vi "RSZVB Set Mixer Delay Constant.vi"(8 "error in (no error)":errorcluster {"code" format="%.0x"}, 9 "Constant Delay (0.0 s)":dbl format="%^.3e", 10 "Channel (1)":i32=1, 11 "VISA session":refnum<visa-resource-name>) -> (0 "error out":errorcluster {"code" format="%.0x"}, 3 "dup VISA session":refnum<visa-resource-name>)   [LabVIEW 2011]
doc: "Defines a constant mixer delay value, to be used as a reference for a mixer delay measurement calibration.\n\nRemote-control command(s):\n[SENSe<Ch>:]FREQuency:MDELay:CDELay"
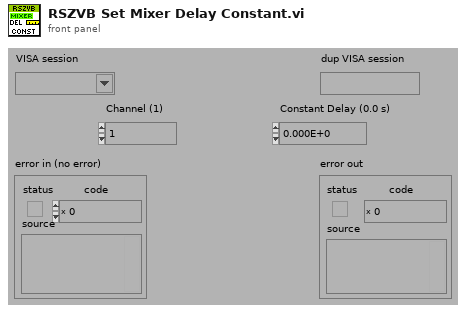
[diagram p1: front panel]
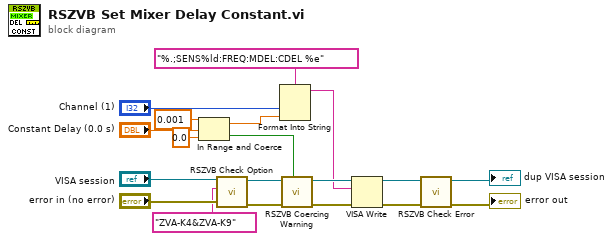
[diagram p0: block diagram]
diagram:
  n1 = In Range and Coerce(upper limit=0.001, x="Constant Delay (0.0 s)", lower limit=0.0) -> (coerced(x)=w8:dbl, In Range?=w9:bool)
  n2 = call "RSZVB Check Option.vi"("error in (no error)"="error in (no error)", "Options"="ZVA-K4&ZVA-K9", "VISA session"="VISA session") -> ("error out"=w11:errorcluster, "dup VISA session"=w10:refnum<visa-resource-name>)  [unwired: 7 in]
  n3 = Format Into String(format string="%.;SENS%ld:FREQ:MDEL:CDEL %e", "Channel (1)", w8) -> (resulting string=w5:string)  [unwired: 2 in, 1 out]
  n4 = call "RSZVB Coercing Warning.vi"("In Range?"=w9, "error in (no error)"=w11, "VISA session"=w10) -> ("error out"=w7:errorcluster, "dup VISA session"=w6:refnum<visa-resource-name>)  [unwired: 7 in]
  n5 = VISA Write(VISA resource name=w6, write buffer=w5, error in (no error)=w7) -> (VISA resource name out=w3:refnum<visa-resource-name>, error out=w4:errorcluster)  [unwired: 1 out]
  n6 = call "RSZVB Check Error.vi"("error in (no error)"=w4, "VISA session"=w3) -> ("error out"=→"error out":errorcluster, "dup VISA session"=→"dup VISA session":refnum<visa-resource-name>)  [unwired: 8 in]
